vi "Proceed.vi"(7 "component is ready (Y)":bool=TRUE, 8 "error in (no error)":errorcluster, 10 "ProceedMessage":refnum<class "ProceedMessage.lvclass">, 11 "ExampleClassA in":refnum<class "ExampleClassA.lvclass">) -> (0 "error out":errorcluster, 2 "all observers are ready?":bool, 3 "ExampleClassA out":refnum<class "ExampleClassA.lvclass">)   [LabVIEW 2012, in "ExampleClassA.lvclass"]
doc: "The Proceed method is used to check if your component is ready. Also it checks if the observers are ready. When the observers and the component are ready, it sends the proceed to its observee. If it's the highest observee, it distributes a stop command."
uses:
  ExampleClassA.lvclass
  <vilib>/Distrio/Murmex/ProceedMessage/ProceedMessage.lvclass
  ExampleClassA.lvclass/ExampleClassA.ctl
  <vilib>/Distrio/Murmex/Murmex/Murmex.lvclass
panel:
  # "This method is called when the PROCEED\ntrigger is sent. \n\nOverride this method when your component needs to\nrespond to this trigger. \n\nCall parent for proper implementation"
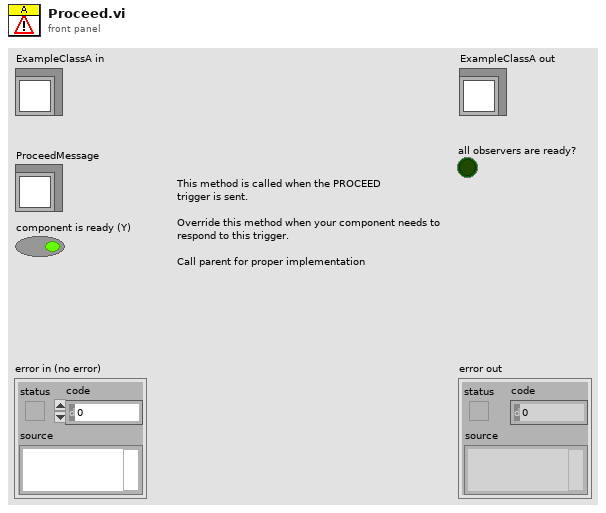
[diagram p1: front panel]
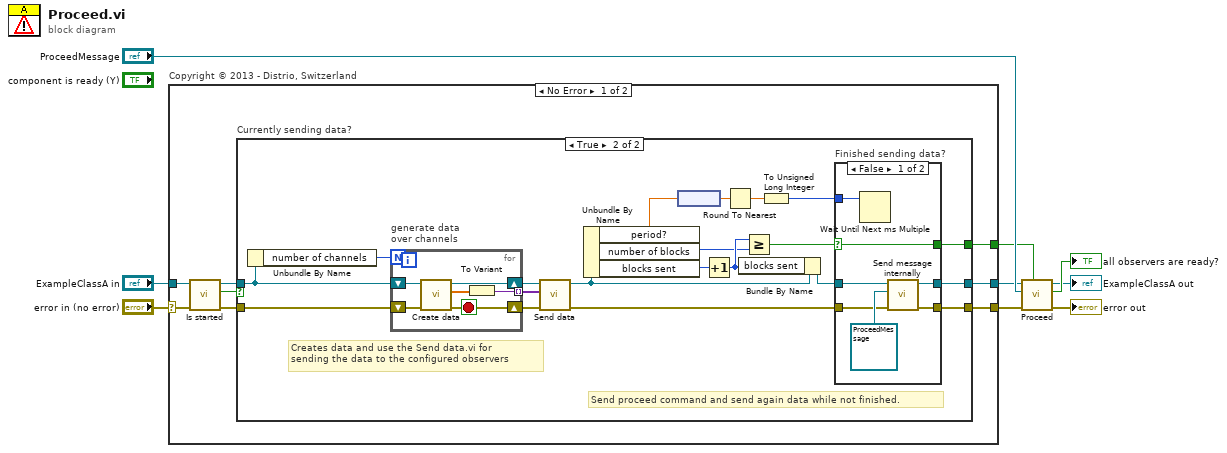
[diagram p0: block diagram]
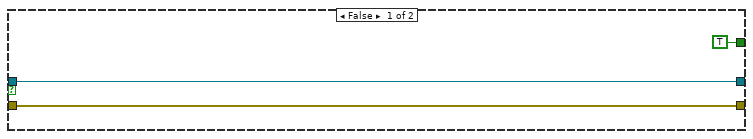
[diagram p2: hidden frame]
diagram:
  n1 = case "Copyright © 2013 - Distrio, Switzerland" shown="No Error" "error in (no error)" {
    selector: "error in (no error)" -> [w17 w58]
    tunnel: "ExampleClassA in" -> [w16 w57]
    tunnel: [w15 w58] -> w3
    tunnel: [w14 w57] -> w2
    tunnel: [w10 _] -> w1
    frame No Error {
      n2 = call <vilib>:"Is started.vi"("error in (no error)"=w17, "Murmex in"=w16) -> ("error out"=w13:errorcluster, "started?"=w11:bool, "Murmex out"=w12:refnum<class "ExampleClassA.lvclass">)  [unwired: 7 in]
      n3 = case "Currently sending data?" shown="True" w11 {
        tunnel: w13 -> [w19 w27]
        tunnel: w12 -> [w20 w30]
        tunnel: [w19 w24] -> w15
        tunnel: [w20 w22] -> w14
        tunnel: [TRUE w21] -> w10
        frame False {
        }
        frame True {
          # "Send proceed command and send again data while not finished."
          # "Creates data and use the Send data.vi for\nsending the data to the configured observers"
          n4 = Unbundle By Name(w30) -> ("number of channels"=w29:i32)
          n5 = for "generate data\nover channels" {
            N: w29 -> [_]
            shift-right: [w46] -> w40
            shift-left: w30 -> [w44]
            shift-right: [w43] -> w26
            shift-left: w27 -> [w45]
            tunnel: [w41] -> w28 mode=indexing
            stop <- w43 stop-if-true
            n6 = call "Create data.vi"("error in (no error)"=w45, "Example Class A in"=w44) -> ("error out"=w43:errorcluster, "Graph"=w42:dbl[], "Example Class A out"=w46:refnum<class "ExampleClassA.lvclass">)  [unwired: 7 in]
            n7 = To Variant(anything=w42) -> (Variant=w41:variant)
          }
          n8 = call <vilib>:"Send data.vi"("error in (no error)"=w26, "data (channels array)"=w28, "Murmex in"=w40) -> ("error out"=w25:errorcluster, "Murmex out"=w35:refnum<class "ExampleClassA.lvclass">)  [unwired: 7 in]
          n9 = Unbundle By Name(w35) -> ("period?"=w39:dbl[unit], "number of blocks"=w32:i32, "blocks sent"=w34:i32)
          n10 = node(w39) -> (w38:dbl)
          n11 = Increment(x=w34) -> (x+1=w33:i32)
          n12 = Round To Nearest(number=w38) -> (nearest integer value=w37:dbl)
          n13 = Bundle By Name(cluster=w35, "blocks sent"=w33) -> (w23:refnum<class "ExampleClassA.lvclass">)
          n14 = Greater Or Equal?(x=w33, y=w32) -> (x >= y?=w31:bool)
          n15 = To Unsigned Long Integer(number=w37) -> (unsigned 32bit integer=w36:u32)
          n16 = case "Finished sending data?" shown="False" w31 {
            selector: w31 -> [w47 w54]
            tunnel: w25 -> [w50 w56]
            tunnel: w36 -> [w53 _]
            tunnel: [w49 w56] -> w24
            tunnel: w23 -> [w52 w55]
            tunnel: [w48 w55] -> w22
            tunnel: [w47 w54] -> w21
            frame False {
              n17 = Wait Until Next ms Multiple(millisecond multiple=w53) -> ()  [unwired: 1 out]
              n18 = call <vilib>:"Send message internally.vi"("error in (no error)"=w50, "Message"=refnum<class "ProceedMessage.lvclass"> refnum ("ProceedMessage"), "Murmex in"=w52) -> ("error out"=w49:errorcluster, "Murmex out"=w48:refnum<class "ExampleClassA.lvclass">)  [unwired: 7 in]
            }
            frame True {
            }
          }
        }
      }
    }
    frame Error {
    }
  }
  n19 = call-parent "Proceed.vi"("component is ready (Y)"=w1, "error in (no error)"=w3, "ProceedMessage"="ProceedMessage", "Murmex in"=w2) -> ("error out"=→"error out":errorcluster, "all observers are ready?"=→"all observers are ready?":bool, "Murmex out"=→"ExampleClassA out":refnum<class "ExampleClassA.lvclass">)  [unwired: 5 in]
